vi "Enable Interrupts.vi"(8 "error in (no error)":errorcluster, 11 "BME_DG_System in":refnum<class "BME_DG_System.lvclass">) -> (0 "error out":errorcluster, 3 "BME_DG_System out":refnum<class "BME_DG_System.lvclass">)   [LabVIEW 2009, in "POLARIS BME DG.lvlib" / "BME_DG_System.lvclass"]
uses:
  BME_DG_System.lvclass
  BME_DG_System.lvclass/BME_DG_System.ctl
  BME_DG_Base/BME_DG_Base.lvclass
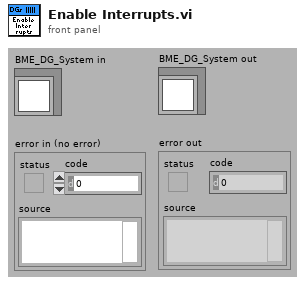
[diagram p1: front panel]
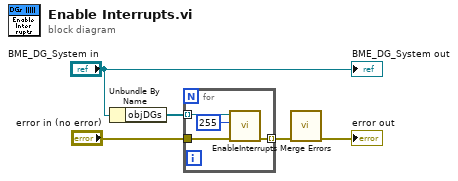
[diagram p0: block diagram]
diagram:
  n1 = Unbundle By Name("BME_DG_System in") -> ("objDGs"=w2:refnum<class "BME_DG_Base.lvclass">[])
  n2 = for {
    tunnel: w2 -> [w9] mode=indexing
    tunnel: "error in (no error)" -> [w8]
    tunnel: [w7] -> w1 mode=indexing
    n3 = call-dynamic "EnableInterrupts.vi"("error in (no error)"=w8, "Interrupt Mask"=u32 255, "BME_DG_Base in"=w9) -> ("error out"=w7:errorcluster)  [unwired: 7 in, 1 out]
  }
  n4 = call <vilib>:"Merge Errors.vi"("error array in"=w1) -> ("error out"=→"error out":errorcluster)  [unwired: 6 in]
  "BME_DG_System out" <- "BME_DG_System in"
